vi "Read commandID.vi"(11 "CommandConstruction in":refnum<class "CommandConstruction.lvclass">) -> (2 "commandID":i32=1 min=0 max=31, 3 "CommandConstruction out":refnum<class "CommandConstruction.lvclass">)   [LabVIEW 2016, in "CommandConstruction.lvclass"]
uses:
  CommandConstruction.lvclass
  CommandConstruction.lvclass/CommandConstruction.ctl
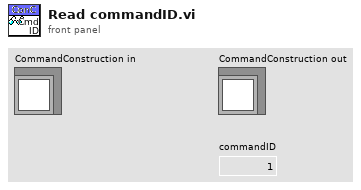
[diagram p1: front panel]
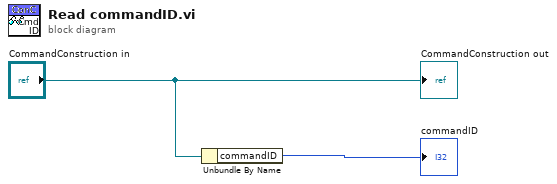
[diagram p0: block diagram]
diagram:
  n1 = Unbundle By Name("CommandConstruction in") -> ("commandID"=→"commandID":i32)
  "CommandConstruction out" <- "CommandConstruction in"
